vi "Acquisition Status.vi"(8 "error in (no error)":errorcluster, 10 "Timeout (10000 ms)":u32=10000, 11 "VISA resource name":refnum<visa-resource-name>) -> (0 "error out":errorcluster, 2 "Acquisition Complete?":bool, 3 "VISA resource name out":refnum<visa-resource-name>)   [LabVIEW 2021, in "Agilent 6000 Series.lvlib"]
doc: "This VI shows the status of the data acquisition process.\n\nNotes:\n(1) This VI does not check the instrument status. Typically, you call this VI only in a sequence of calls to other low-level driver VIs. The sequence performs one operation. You use the low-level VIs to optimize one or more aspects of interaction with the instrument. If you want to check the instrument status, call the ag6000a Error-Query.vi at the conclusion of the sequence."
uses:
  Agilent 6000 Series.lvlib
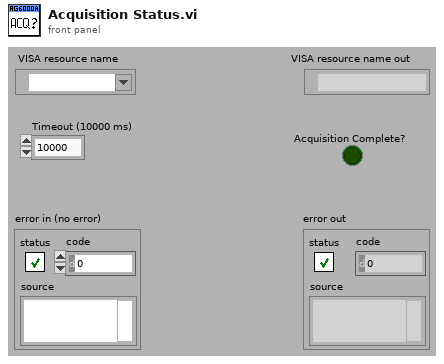
[diagram p1: front panel]
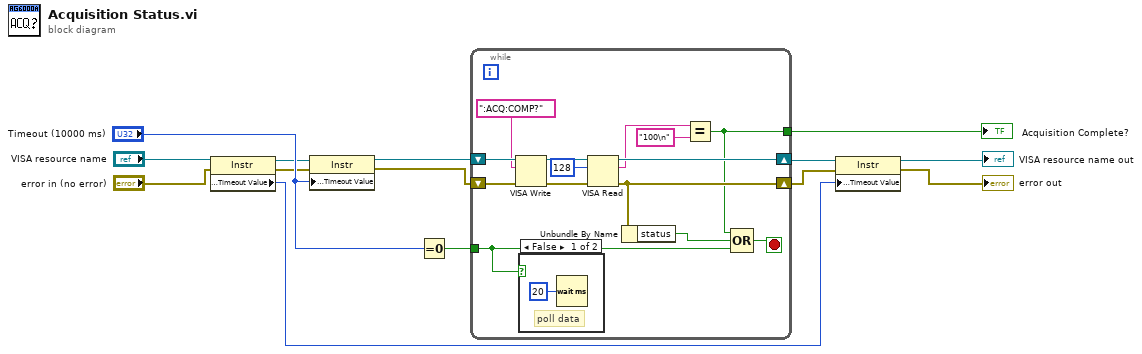
[diagram p0: block diagram]
diagram:
  n1 = property on="Property Node" class="Instr"(reference="VISA resource name", error in="error in (no error)") -> (reference out=w8:refnum<visa-resource-name>, error out=w7:errorcluster, "General Settings:Timeout Value"=w4:u32)
  n2 = property on="Property Node" class="Instr"(reference=w8, error in=w7, "General Settings:Timeout Value"="Timeout (10000 ms)") -> (reference out=w13:refnum<visa-resource-name>, error out=w12:errorcluster)
  n3 = Equal To 0?(x="Timeout (10000 ms)") -> (x = 0?=w14:bool)
  n4 = while {
    tunnel: w14 -> [w16]
    shift-right: [w24] -> w5
    shift-left: w13 -> [w28]
    shift-right: [w21] -> w6
    shift-left: w12 -> [w27]
    tunnel: [w15] -> w3
    stop <- w20 stop-if-true
    n5 = VISA Write(VISA resource name=w28, write buffer=":ACQ:COMP?", error in (no error)=w27) -> (VISA resource name out=w23:refnum<visa-resource-name>, error out=w25:errorcluster)  [unwired: 1 out]
    n6 = case shown="False" w16 {
      frame False {
        # "poll data"
        n7 = Wait (ms)(milliseconds to wait=u32 20) -> ()  [unwired: 1 out]
      }
      frame True {
      }
    }
    n8 = VISA Read(VISA resource name=w23, byte count=u32 128, error in (no error)=w25) -> (VISA resource name out=w24:refnum<visa-resource-name>, read buffer=w18:string, error out=w21:errorcluster)  [unwired: 1 out]
    n9 = Unbundle By Name(w21) -> ("status"=w19:bool)
    n10 = Equal?(x=w18, y="100\n") -> (x = y?=w15:bool)
    n11 = Compound Arithmetic op=OR(w15, w19, w16) -> (w20:bool)
  }
  "Acquisition Complete?" <- w3
  n12 = property on="Property Node" class="Instr"(reference=w5, error in=w6, "General Settings:Timeout Value"=w4) -> (reference out=→"VISA resource name out":refnum<visa-resource-name>, error out=→"error out":errorcluster)
